vi "ReadWrite - Settings.vi"(0 "Data (out) in":T1, 2 "Action":enum16{"Read", "Write"}(ring), 11 "error in (no error)":errorcluster) -> (4 "Data (out) out":T1, 15 "error out":errorcluster)   [LabVIEW 2020]
uses:
  TypeDefs/Data.ctl
  <vilib>/Utility/config.llb/Read Key (Boolean).vi
  <vilib>/Utility/config.llb/Read Key (Path).vi
  <vilib>/Utility/config.llb/Write Key (Boolean).vi
  <vilib>/Utility/config.llb/Write Key (Path).vi
  <vilib>/Utility/config.llb/NI_LVConfig.lvlib
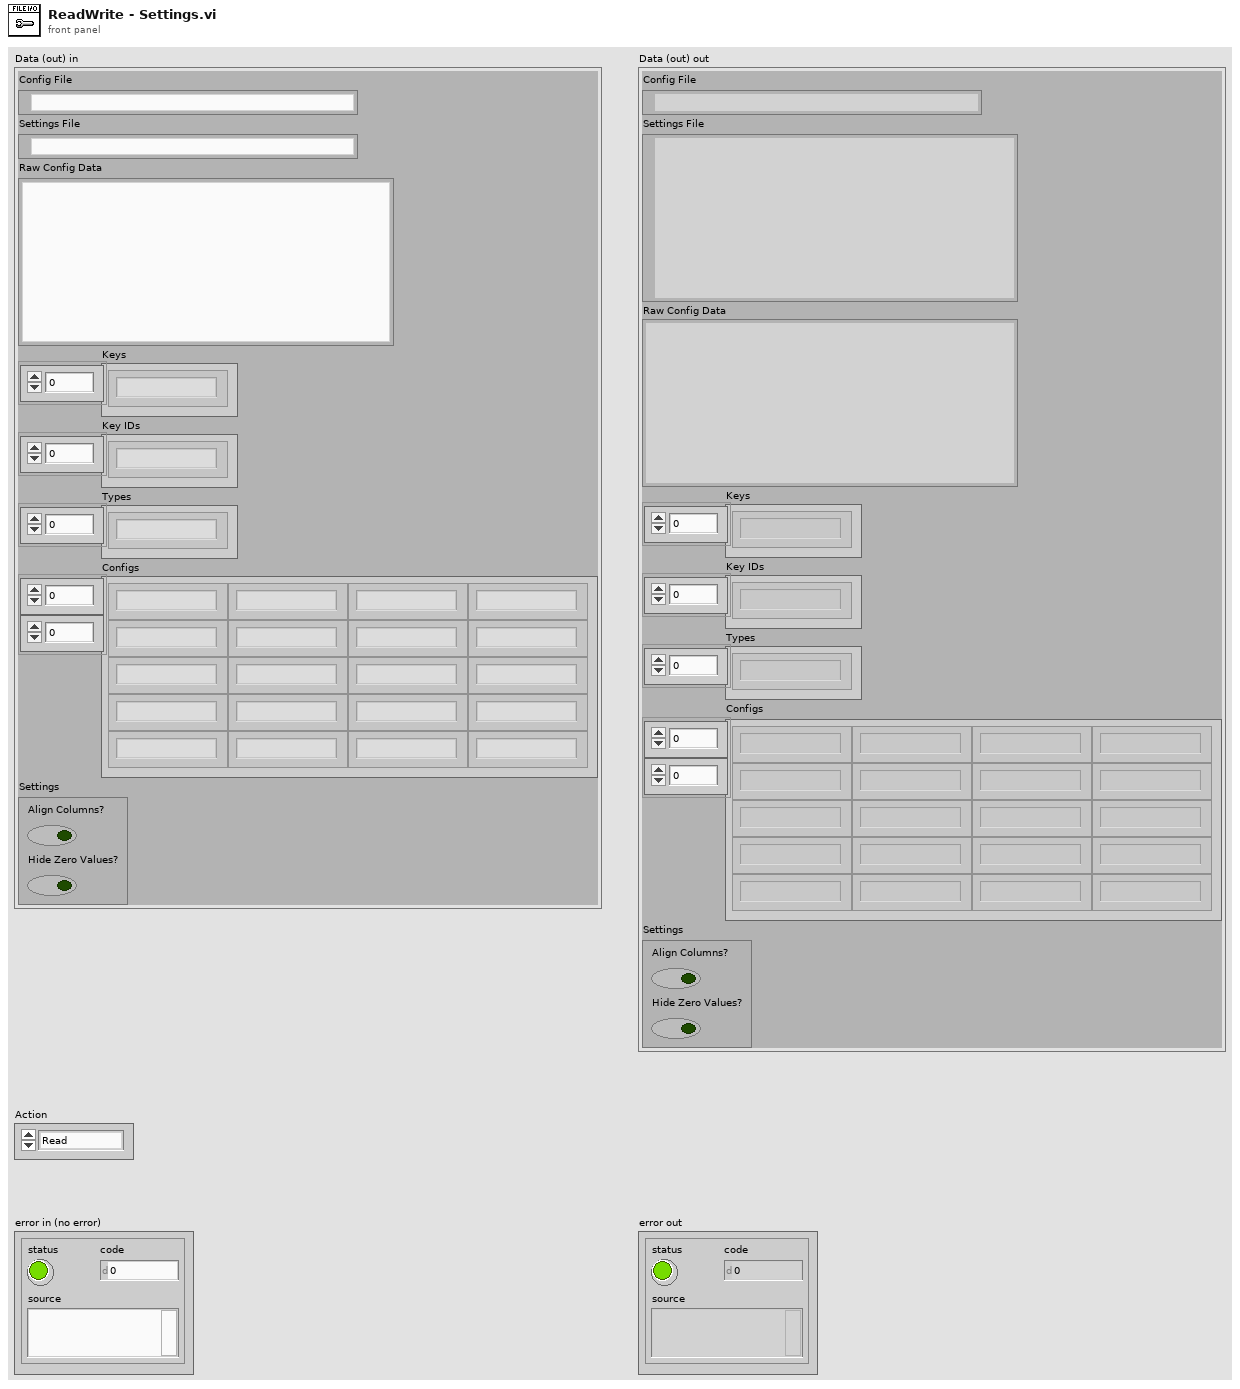
[diagram p1: front panel]
types:
  T1 = typedef "Data.ctl" = cluster{"Config File":path, "Settings File":path, "Raw Config Data":string, "Keys":string[], "Key IDs":string[], "Types":string[], "Configs":string[][], "Settings":cluster{"Align Columns?":bool, "Hide Zero Values?":bool}}
  T2 = typedef "NI_LVConfig.lvlib/Config Data RefNum.ctl" = refnum<k1>
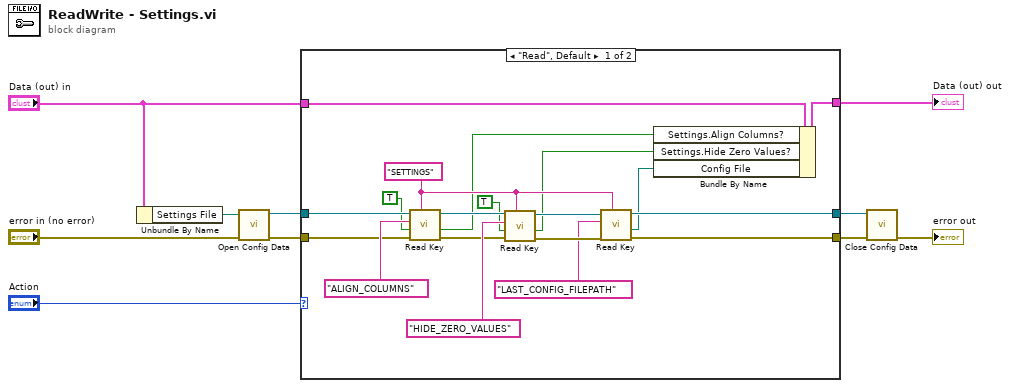
[diagram p0: block diagram]
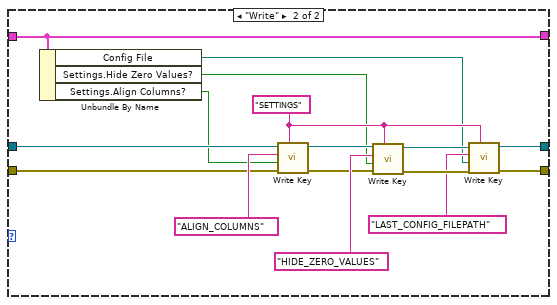
[diagram p2: hidden frame]
diagram:
  n1 = Unbundle By Name("Data (out) in") -> ("Settings File"=w10:path)
  n2 = call <vilib>:"Open Config Data.vi"("error in (no error)"="error in (no error)", "configuration file path"=w10) -> ("error out"=w4:errorcluster, "refnum"=w1:T2)  [unwired: 7 in, 1 out]
  n3 = case shown="\"Read\", Default" "Action" {
    tunnel: w1 -> [w29 w45]
    tunnel: [w21 w37] -> w2
    tunnel: [w20 w36] -> w3
    tunnel: w4 -> [w19 w35]
    tunnel: "Data (out) in" -> [w14 w33]
    tunnel: [w13 w33] -> w8
    frame "Read", Default {
      w24 = "SETTINGS" ("section")
      n4 = call-poly <vilib>:"Read Key.vi"("section"=w24, "error in (no error)"=w19, "default value"=TRUE, "key"="ALIGN_COLUMNS", "refnum"=w29) -> ("error out"=w18:errorcluster, "value"=w17:bool, "refnum out"=w28:T2)  [unwired: 3 in, 1 out]
      n5 = call-poly <vilib>:"Read Key.vi"("section"=w24, "error in (no error)"=w18, "default value"=TRUE, "key"="HIDE_ZERO_VALUES", "refnum"=w28) -> ("error out"=w25:errorcluster, "value"=w16:bool, "refnum out"=w26:T2)  [unwired: 3 in, 1 out]
      n6 = call-poly <vilib>:"Read Key.vi"("section"=w24, "error in (no error)"=w25, "key"="LAST_CONFIG_FILEPATH", "refnum"=w26) -> ("error out"=w21:errorcluster, "value"=w15:path, "refnum out"=w20:T2)  [unwired: 4 in, 1 out]
      n7 = Bundle By Name(cluster=w14, "Settings.Align Columns?"=w17, "Settings.Hide Zero Values?"=w16, "Config File"=w15) -> (w13:T1)
    }
    frame "Write" {
      w40 = "SETTINGS" ("section")
      n8 = Unbundle By Name(w33) -> ("Config File"=w32:path, "Settings.Hide Zero Values?"=w31:bool, "Settings.Align Columns?"=w30:bool)
      n9 = call-poly <vilib>:"Write Key.vi"("section"=w40, "error in (no error)"=w35, "value"=w30, "key"="ALIGN_COLUMNS", "refnum"=w45) -> ("error out"=w34:errorcluster, "refnum out"=w44:T2)  [unwired: 4 in, 1 out]
      n10 = call-poly <vilib>:"Write Key.vi"("section"=w40, "error in (no error)"=w34, "value"=w31, "key"="HIDE_ZERO_VALUES", "refnum"=w44) -> ("error out"=w41:errorcluster, "refnum out"=w42:T2)  [unwired: 4 in, 1 out]
      n11 = call-poly <vilib>:"Write Key.vi"("section"=w40, "error in (no error)"=w41, "value"=w32, "key"="LAST_CONFIG_FILEPATH", "refnum"=w42) -> ("error out"=w37:errorcluster, "refnum out"=w36:T2)  [unwired: 4 in, 1 out]
    }
  }
  "Data (out) out" <- w8
  n12 = call <vilib>:"Close Config Data.vi"("error in (no error)"=w2, "refnum"=w3) -> ("error out"=→"error out":errorcluster)  [unwired: 8 in, 1 out]
